vi "Read.Pcap.File.vi"(10 "PCap File":string, 11 "Path":path) -> (1 "Records":T1[](array[typedef]) {"ts_sec" format="%.0x"; "ts_usec" format="%.0x"; "incl_len" format="%.0x"; "orig_len" format="%.0x"; "payload" format="%.0x"}, 2 "Global\nHeader":T2={"magic_number"=3569595041, "version_major"=512, "version_minor"=1024, "thiszone"=0, "sigfigs"=0, "snap_len"=1024, "network"=16777216} {"magic_number" format="%.0x"; "version_major" format="%.0x"; "version_minor" format="%.0x"; "thiszone" format="%.0x"; "sigfigs" format="%.0x"; "network" format="%.0x"}, 3 "Swap?":bool)   [LabVIEW 2020]
uses:
  global.header.ctl
  record.ctl
panel:
  out "# of Records":i32
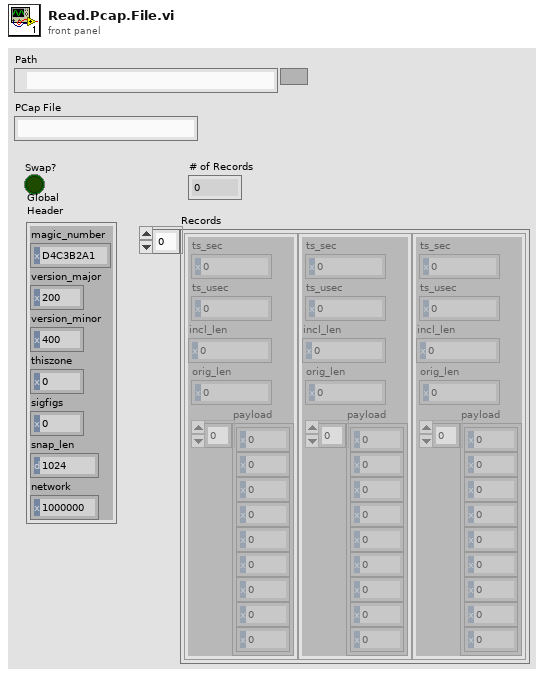
[diagram p1: front panel]
types:
  T1 = typedef "record.ctl" = cluster{"ts_sec":u32, "ts_usec":u32, "incl_len":u32, "orig_len":u32, "payload":u8[]}
  T2 = typedef "global.header.ctl" = cluster{"magic_number":u32, "version_major":u16, "version_minor":u16, "thiszone":u32, "sigfigs":u32, "snap_len":u32, "network":u32}
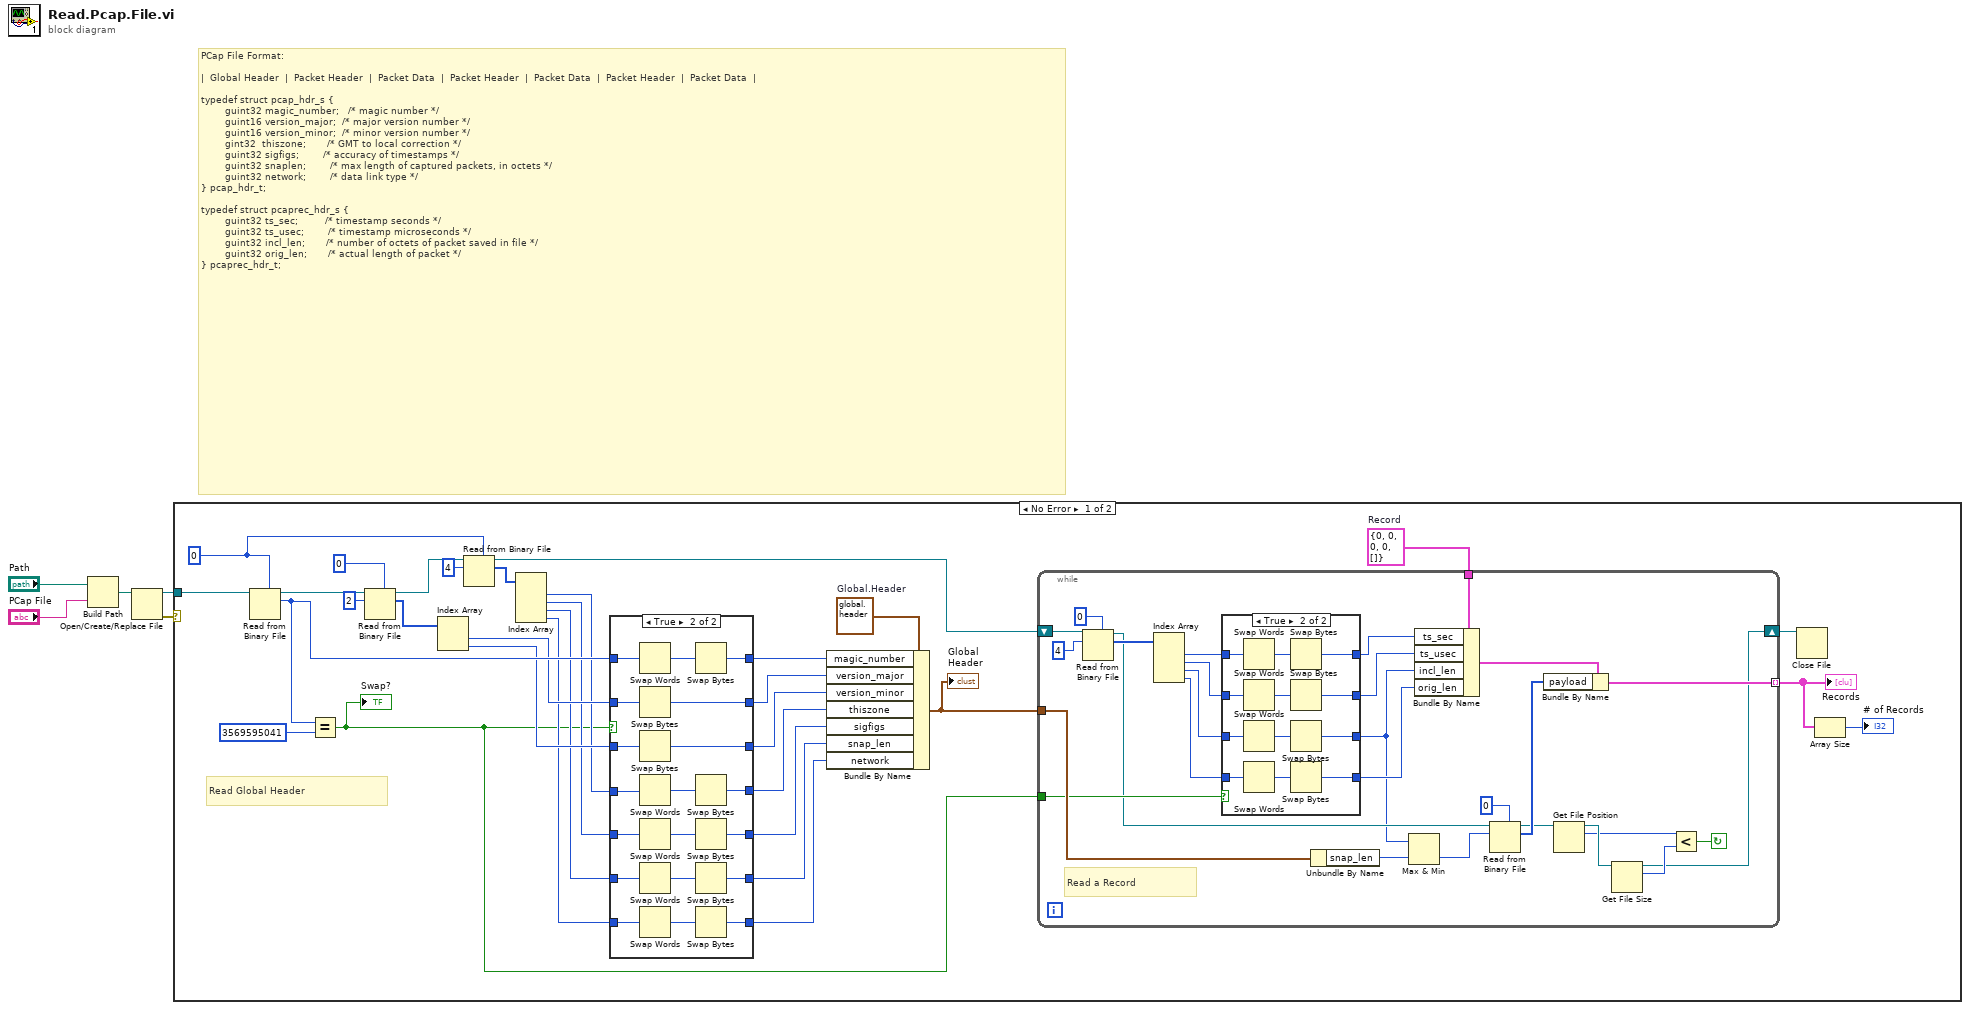
[diagram p0: block diagram]
diagram:
  # "PCap File Format:\n\n|  Global Header  |  Packet Header  |  Packet Data  |  Packet Header  |  Packet Data  |  Packet Header  |  Packet Data  |\n\ntypedef struct pcap_hdr_s {\n        guint32 magic_number;   /* magic number */\n        guint16 version_major;  /* major version number */\n        guint16 version_minor;  /* minor version number */\n        gint32  thiszone;       /* GMT to local correction */\n        guint32 sigfigs;        /* accuracy of timestamps */\n        guint32 snaplen;        /* max length of captured packets, in octets */\n        guint32 network;        /* data link type */\n} pcap_hdr_t;\n\ntypedef struct pcaprec_hdr_s {\n        guint32 ts_sec;         /* timestamp seconds */\n        guint32 ts_usec;        /* timestamp microseconds */\n        guint32 incl_len;       /* number of octets of packet saved in file */\n        guint32 orig_len;       /* actual length of packet */\n} pcaprec_hdr_t;"
  n1 = Build Path(base path="Path", name or relative path="PCap File") -> (appended path=w3:path)
  n2 = Open/Create/Replace File(file path (use dialog)=w3) -> (refnum out=w1:refnum<file>, error out=w2:errorcluster)  [unwired: 5 in, 1 out]
  n3 = case shown="No Error" w2 {
    tunnel: w1 -> [w37 _]
    frame No Error {
      w6 = T1 {"ts_sec"=0, "ts_usec"=0, "incl_len"=0, "orig_len"=0, "payload"=[]}  # Record
      w7 = T2 {"magic_number"=3569595041, "version_major"=512, "version_minor"=1024, "thiszone"=0, "sigfigs"=0, "snap_len"=1024, "network"=16777216}  # Global.Header
      w30 = u32 0
      # "Read Global Header"
      n4 = Read from Binary File(5:w30, 11:w37) -> (2:w27:u32, 3:w34:refnum<file>)  [unwired: 4 in, 2 out]
      n5 = Equal?(x=w27, y=u32 3569595041) -> (x = y?=w9:bool)
      "Swap?" <- w9
      n6 = Read from Binary File(5:u16 0, 10:2 ("count (1)"), 11:w34) -> (2:w32:u16[], 3:w31:refnum<file>)  [unwired: 3 in, 2 out]
      n7 = Index Array(array=w32) -> (element #1=w25:u16, element #2=w24:u16)  [unwired: 2 in]
      n8 = Read from Binary File(5:w30, 10:4 ("count (1)"), 11:w31) -> (2:w28:u32[], 3:w13:refnum<file>)  [unwired: 3 in, 2 out]
      n9 = Index Array(array=w28) -> (element #1=w21:u32, element #2=w19:u32, element #3=w18:u32, element #4=w17:u32)  [unwired: 4 in]
      n10 = case shown="True" w9 {
        tunnel: w27 -> [w88 w107]
        tunnel: [w88 w105] -> w26
        tunnel: w25 -> [w87 w104]
        tunnel: w24 -> [w86 w103]
        tunnel: [w87 w102] -> w23
        tunnel: [w86 w101] -> w22
        tunnel: w21 -> [w85 w96]
        tunnel: [w85 w95] -> w20
        tunnel: w19 -> [w84 w94]
        tunnel: w18 -> [w83 w93]
        tunnel: w17 -> [w82 w92]
        tunnel: [w84 w91] -> w16
        tunnel: [w83 w90] -> w15
        tunnel: [w82 w89] -> w14
        frame False {
        }
        frame True {
          n11 = Swap Words(1:w107) -> (0:w106:u32)
          n12 = Swap Bytes(anything=w104) -> (byte swapped=w102:u16)
          n13 = Swap Bytes(anything=w103) -> (byte swapped=w101:u16)
          n14 = Swap Words(1:w96) -> (0:w100:u32)
          n15 = Swap Words(1:w94) -> (0:w99:u32)
          n16 = Swap Words(1:w93) -> (0:w98:u32)
          n17 = Swap Words(1:w92) -> (0:w97:u32)
          n18 = Swap Bytes(anything=w106) -> (byte swapped=w105:u32)
          n19 = Swap Bytes(anything=w100) -> (byte swapped=w95:u32)
          n20 = Swap Bytes(anything=w99) -> (byte swapped=w91:u32)
          n21 = Swap Bytes(anything=w98) -> (byte swapped=w90:u32)
          n22 = Swap Bytes(anything=w97) -> (byte swapped=w89:u32)
        }
      }
      n23 = Bundle By Name(cluster=w7, "magic_number"=w26, "version_major"=w23, "version_minor"=w22, "thiszone"=w20, "sigfigs"=w16, "snap_len"=w15, "network"=w14) -> (w8:T2)
      "Global\nHeader" <- w8
      n24 = while {
        tunnel: w6 -> [w61]
        tunnel: [w52] -> w11 mode=indexing
        shift-right: [w51] -> w12
        shift-left: w13 -> [w65]
        tunnel: w8 -> [w49]
        tunnel: w9 -> [w47]
        stop <- w53 continue-if-true
        # "Read a Record"
        n25 = Read from Binary File(5:u32 0 ("count (1)"), 10:4 ("count (1)"), 11:w65) -> (2:w62:u32[], 3:w44:refnum<file>)  [unwired: 3 in, 2 out]
        n26 = Index Array(array=w62) -> (element #1=w46:u32, element #2=w43:u32, element #3=w42:u32, element #4=w41:u32)  [unwired: 4 in]
        n27 = case shown="True" w47 {
          tunnel: w46 -> [w69 w81]
          tunnel: [w69 w79] -> w45
          tunnel: w43 -> [w68 w78]
          tunnel: w42 -> [w67 w76]
          tunnel: w41 -> [w66 w75]
          tunnel: [w68 w72] -> w40
          tunnel: [w67 w71] -> w38
          tunnel: [w66 w70] -> w39
          frame False {
          }
          frame True {
            n28 = Swap Words(1:w81) -> (0:w80:u32)
            n29 = Swap Words(1:w78) -> (0:w77:u32)
            n30 = Swap Words(1:w76) -> (0:w73:u32)
            n31 = Swap Words(1:w75) -> (0:w74:u32)
            n32 = Swap Bytes(anything=w80) -> (byte swapped=w79:u32)
            n33 = Swap Bytes(anything=w77) -> (byte swapped=w72:u32)
            n34 = Swap Bytes(anything=w73) -> (byte swapped=w71:u32)
            n35 = Swap Bytes(anything=w74) -> (byte swapped=w70:u32)
          }
        }
        n36 = Unbundle By Name(w49) -> ("snap_len"=w48:u32)
        n37 = Max & Min(x=w38, y=w48) -> (min(x,y)=w50:u32)  [unwired: 1 out]
        n38 = Bundle By Name(cluster=w61, "ts_sec"=w45, "ts_usec"=w40, "incl_len"=w38, "orig_len"=w39) -> (w59:T1)
        n39 = Read from Binary File(5:u8 0 ("count (1)"), 10:w50, 11:w44) -> (2:w58:u8[], 3:w57:refnum<file>)  [unwired: 3 in, 2 out]
        n40 = Bundle By Name(cluster=w59, "payload"=w58) -> (w52:T1)
        n41 = Get File Position(7:w57) -> (2:w55:i64, 3:w56:refnum<file>)  [unwired: 1 in, 1 out]
        n42 = Get File Size(file=w56) -> (refnum out=w51:refnum<file>, size (in bytes)=w54:i64)  [unwired: 1 in, 1 out]
        n43 = Less?(x=w55, y=w54) -> (x < y?=w53:bool)
      }
      "Records" <- w11
      n44 = Close File(refnum=w12) -> ()  [unwired: 1 in, 2 out]
      n45 = Array Size(array=w11) -> (size(s)=→"# of Records":i32)
    }
    frame Error {
    }
  }
